vi "RPopLPush.vi"(0 "reference in":refnum<class "Redis.lvclass">, 5 "Source":string, 9 "Destination":string, 11 "Error In":errorcluster) -> (4 "reference out":refnum<class "Redis.lvclass">, 8 "Data":T1, 15 "Error Out":errorcluster)   [LabVIEW 2020, in "Redis.lvclass"]
doc: "<b>RPOPLPUSH</b>\n\nAtomically returns and removes the last element (tail) of the list stored at source, and pushes the element at the first element (head) of the list stored at destination.\n\nFor example: consider source holding the list a,b,c, and destination holding the list x,y,z. Executing RPOPLPUSH results in source holding a,b and destination holding c,x,y,z.\n\nIf source does not exist, the value nil is returned and no operation is performed. If source and destination are the same, the operation is equivalent to removing the last element from the list and pushing it as first element of the list, so it can be considered as a list rotation command."
uses:
  Redis.lvclass
  ReplyDataTypeEnum.ctl
  RedisDataType.ctl
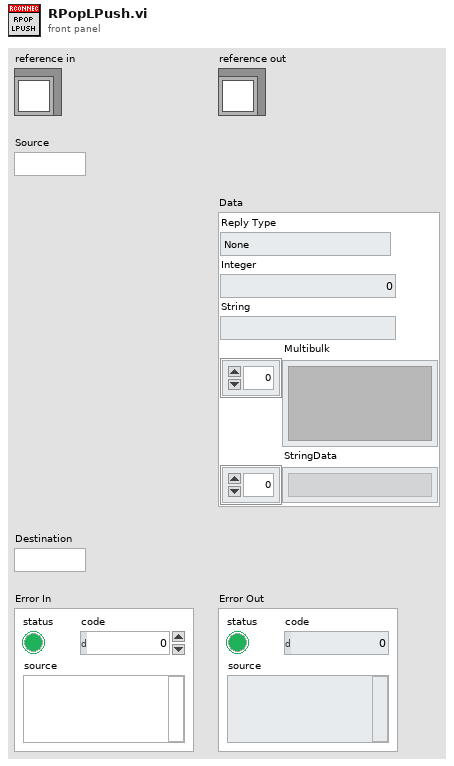
[diagram p1: front panel]
types:
  T1 = typedef "Redis.lvclass/RedisDataType.ctl" = cluster{"Reply Type":T2, "Integer":i64, "String":string, "Multibulk":variant[], "StringData":string[]}
  T2 = typedef "Redis.lvclass/ReplyDataTypeEnum.ctl" = enum16{"None", "Error", "Status", "Nil", "Integer", "String", "Multibulk"}
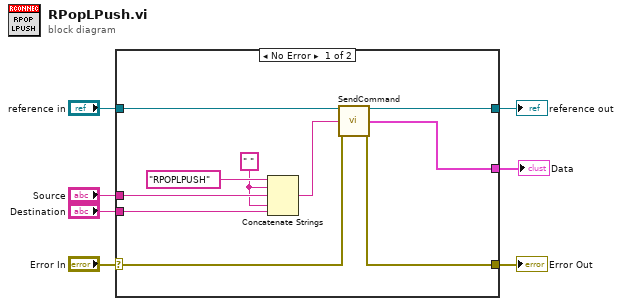
[diagram p0: block diagram]
diagram:
  n1 = case shown="No Error" "Error In" {
    selector: "Error In" -> [w15 w19]
    tunnel: [w14 w19] -> w6
    tunnel: [w17 w18] -> w4
    tunnel: "reference in" -> [w16 w18]
    tunnel: [w13 _] -> w3
    tunnel: "Source" -> [w11 _]
    tunnel: "Destination" -> [w8 _]
    frame No Error {
      w9 = " "
      n2 = Concatenate Strings("RPOPLPUSH", w9, w11, w9, w8) -> (w10:string)
      n3 = call "SendCommand.vi"("reference in"=w16, "Command"=w10, "Error In"=w15) -> ("reference out"=w17:refnum<class "Redis.lvclass">, "Data"=w13:T1, "Error Out"=w14:errorcluster)  [unwired: 10 in]
    }
    frame Error {
    }
  }
  "Error Out" <- w6
  "reference out" <- w4
  "Data" <- w3
